vi "_Main.vi"   [LabVIEW 2017, in "VisionSystem.lvlib"]
uses:
  VisionSystem.lvlib
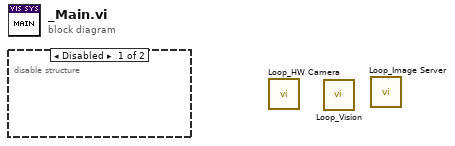
[diagram p0: block diagram]
diagram:
  n1 = disable-structure shown="Disabled" {
    frame Disabled {
    }
    frame Enabled {
    }
  }
  n2 = call "Loop_HW Camera.vi"() -> ()  [unwired: 12 in]
  n3 = call "Loop_Vision.vi"() -> ()  [unwired: 12 in]
  n4 = call "Loop_Image Server.vi"() -> ()  [unwired: 12 in]
